vi "Queue Last Ack.vi"(10 "Queue jettl":refnum<class "Queue jettl.lvclass">, 11 "Base Queue jettl in":refnum<class "Base Queue jettl.lvclass">) -> (3 "Base Queue jettl out":refnum<class "Base Queue jettl.lvclass">)   [LabVIEW 2021, in "jettl.lvlib" / "Base Queue jettl.lvlib" / "Base Queue jettl.lvclass"]
uses:
  Base Queue jettl.lvclass
  Queue jettl/Queue jettl.lvclass
  Msg Strategy/Msg Strategy.lvclass
  Base Queue jettl.lvclass/Base Queue jettl.ctl
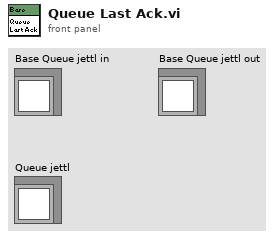
[diagram p1: front panel]
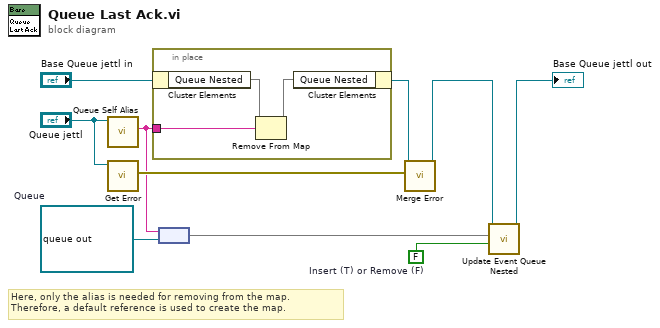
[diagram p0: block diagram]
diagram:
  w1 = refnum<data-value> refnum  # Queue
  w7 = FALSE  # Insert (T) or Remove (F)
  # "Here, only the alias is needed for removing from the map. Therefore, a default reference is used to create the map."
  n1 = call-dynamic "Queue Self Alias.vi"("jettl in"="Queue jettl") -> ("Queue Self Alias"=w3:string)  [unwired: 10 in]
  n2 = call-dynamic "Get Error.vi"("jettl in"="Queue jettl") -> ("Error"=w10:errorcluster)  [unwired: 10 in]
  n3 = in-place {
    in-place-border: w3 -> [w11]
    n4 = in-place-cluster #1("Base Queue jettl in") -> ("Queue Nested"=w12:map{string, refnum<data-value>})
    n5 = Remove From Map(10:w11, 11:w12) -> (3:w13:map{string, refnum<data-value>})  [unwired: 2 out]
    n6 = in-place-cluster #1("Queue Nested"=w13) -> (w9:refnum<class "Base Queue jettl.lvclass">)
  }
  n7 = node(w3, w1) -> (w2:map{string, refnum<data-value>})
  n8 = call-dynamic "Merge Error.vi"("Error"=w10, "Base Queue jettl in"=w9) -> ("Base Queue jettl out"=w6:refnum<class "Base Queue jettl.lvclass">)  [unwired: 9 in]
  n9 = call "Update Event Queue Nested.vi"("Insert (T) or Remove (F)"=w7, "Queue Nested"=w2, "Base Queue jettl in"=w6) -> ("Base Queue jettl out"=→"Base Queue jettl out":refnum<class "Base Queue jettl.lvclass">)  [unwired: 8 in]
